vi "Set Trigger Sense Div.vi"(8 "error in (no error)":errorcluster, 10 "y_scale":dbl, 11 "sense":dbl) -> (0 "error out":errorcluster)   [LabVIEW 2023, in "vmmsolib.lvlib"]
doc: "DLL_API void WINAPI SetTriggerSenseDiv(double sense, double y_scale);"
uses:
  vmmsolib.lvlib
  vmmso.dll
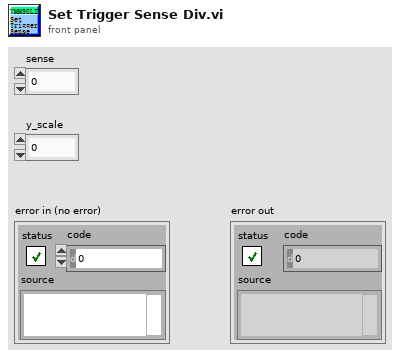
[diagram p1: front panel]
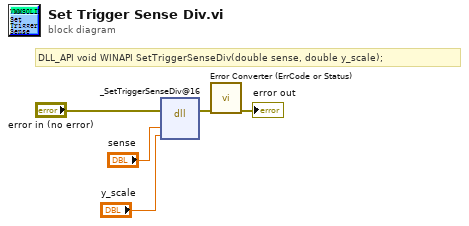
[diagram p0: block diagram]
diagram:
  # "DLL_API void WINAPI SetTriggerSenseDiv(double sense, double y_scale);"
  n1 = dll-call lib="D:/VmMsoSDK/demo-Labview/2023/vmmsolib/vmmso.*" fn="_SetTriggerSenseDiv@16"(error in="error in (no error)", "sense"="sense", "y_scale"="y_scale") -> (error out=w2:errorcluster)  [unwired: 5 in, 1 out]
  n2 = call "Error Converter (ErrCode or Status).vi"("error in (no error)"=w2) -> ("error out"=→"error out":errorcluster)  [unwired: 10 in]
